vi "Insert Start Message.vi"(8 "error in (no error)":errorcluster, 10 "Start Time":timestamp, 11 "AcquistionObject in":refnum<class "AcquistionObject.lvclass">) -> (0 "error out":errorcluster, 3 "AcquistionObject out":refnum<class "AcquistionObject.lvclass">)   [LabVIEW 2014, in "AcquisitionCoreObjects.lvlib" / "AcquistionObject.lvclass"]
uses:
  AcquistionObject.lvclass
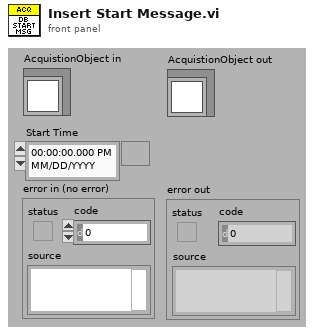
[diagram p1: front panel]
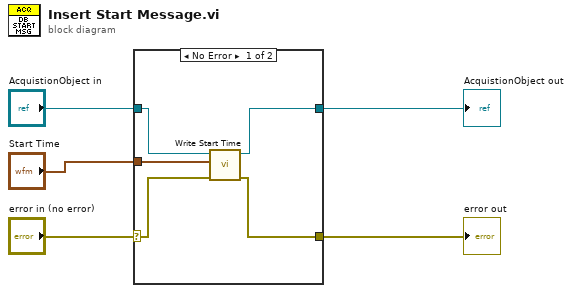
[diagram p0: block diagram]
diagram:
  n1 = case shown="No Error" "error in (no error)" {
    selector: "error in (no error)" -> [w7 w12]
    tunnel: [w6 w12] -> w4
    tunnel: [w8 w11] -> w2
    tunnel: "AcquistionObject in" -> [w9 w11]
    tunnel: "Start Time" -> [w10 _]
    frame No Error {
      n2 = call-dynamic "Write Start Time.vi"("error in (no error)"=w7, "Start Time"=w10, "AcquistionObject in"=w9) -> ("error out"=w6:errorcluster, "AcquistionObject out"=w8:refnum<class "AcquistionObject.lvclass">)  [unwired: 7 in]
    }
    frame Error {
    }
  }
  "error out" <- w4
  "AcquistionObject out" <- w2
